vi "Main.vi"() -> ()   [LabVIEW 2017]
panel:
  out "speed":dbl(knob) scale=0.0..10.0
  out "i":i32
  in  "STATUS":string
  in  "stop":bool
  out "ip":string
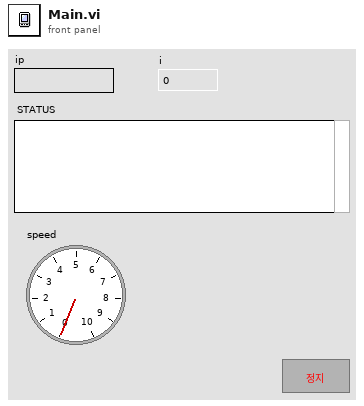
[diagram p1: front panel]
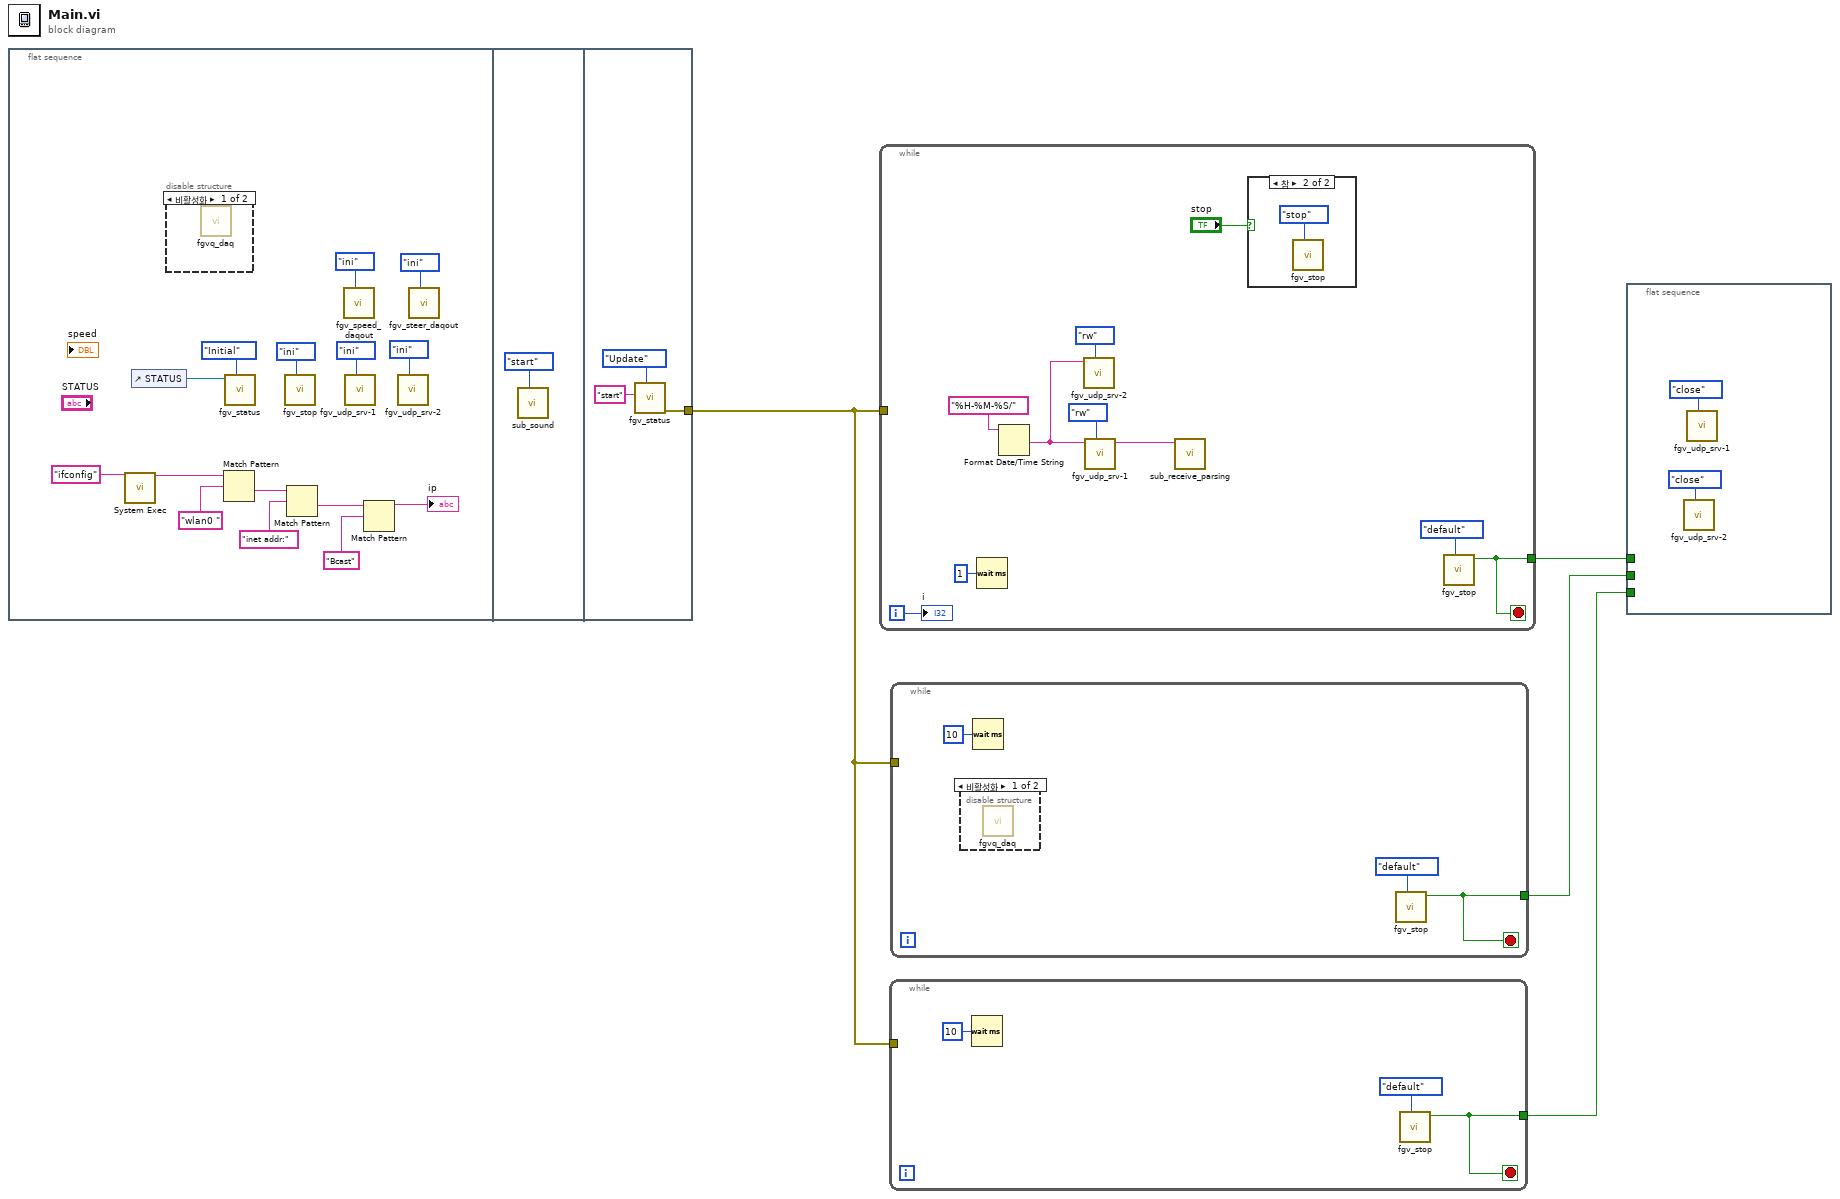
[diagram p0: block diagram]
diagram:
  n1 = flat-sequence {
    tunnel: [w21] -> w1
    frame #0 {
      n2 = call <vilib>:"System Exec.vi"("command line"="ifconfig") -> ("standard output"=w18:string)  [unwired: 7 in, 3 out]
      n3 = control-ref of="STATUS"() -> (w11:refnum<vi>)
      n4 = disable-structure shown="비활성화" {
        frame Disabled {
          n5 = call "fgvq_daq.vi"() -> ()  [unwired: 10 in, 2 out]
        }
        frame Enabled {
        }
      }
      n6 = Match Pattern(string=w18, regular expression="wlan0 ") -> (after substring=w16:string)  [unwired: 1 in, 3 out]
      n7 = call "fgv_status.vi"("Mode"=enum16{"Initial", "Update", "Clear"}."Initial", "System Log"=w11) -> ()  [unwired: 9 in, 1 out]
      n8 = call "fgv_stop.vi"("cmd"=enum16{"default", "ini", "stop"}."ini") -> ()  [unwired: 9 in, 2 out]
      n9 = Match Pattern(string=w16, regular expression="inet addr:") -> (after substring=w14:string)  [unwired: 1 in, 3 out]
      n10 = call "fgv_speed_daqout.vi"("cmd"=enum16{"speed", "close", "ini"}."ini") -> ()  [unwired: 10 in, 1 out]
      n11 = call "fgv_udp_srv-1.vi"("cmd"=enum16{"close", "rw", "ini"}."ini") -> ()  [unwired: 9 in, 2 out]
      n12 = Match Pattern(string=w14, regular expression="Bcast") -> (before substring=→"ip":string)  [unwired: 1 in, 3 out]
      n13 = call "fgv_udp_srv-2.vi"("cmd"=enum16{"close", "rw", "ini"}."ini") -> ()  [unwired: 9 in, 2 out]
      n14 = call "fgv_steer_daqout.vi"("cmd"=enum16{"steer", "close", "ini"}."ini") -> ()  [unwired: 10 in, 1 out]
    }
    frame #1 {
      n15 = call "sub_sound.vi"("cmd"=enum16{"start", "key_lock"}."start") -> ()  [unwired: 10 in, 1 out]
    }
    frame #2 {
      n16 = call "fgv_status.vi"("Mode"=enum16{"Initial", "Update", "Clear"}."Update", "String in"="start") -> ("ERR-OUT"=w21:errorcluster)  [unwired: 9 in]
    }
  }
  n17 = while {
    tunnel: [w26] -> w4
    tunnel: w1 -> [_]
    i -> [w27]
    stop <- w26 stop-if-true
    n18 = Wait (ms)(milliseconds to wait=u32 1 ("대기 시간 (ms)")) -> ()  [unwired: 1 out]
    n19 = Format Date/Time String(time format string (%c)="%H-%M-%S/" ("시간 포맷 문자열 (%c)")) -> (date/time string=w28:string)  [unwired: 2 in]
    n20 = call "fgv_udp_srv-2.vi"("cmd"=enum16{"close", "rw", "ini"}."rw", "data_in"=w28) -> ()  [unwired: 8 in, 2 out]
    n21 = call "fgv_udp_srv-1.vi"("cmd"=enum16{"close", "rw", "ini"}."rw", "data_in"=w28) -> ("data_out"=w24:string)  [unwired: 8 in, 1 out]
    n22 = call "sub_receive_parsing.vi"("data_out 입력"=w24) -> ()  [unwired: 10 in, 1 out]
    n23 = case shown="참" "stop" {
      frame False {
      }
      frame True {
        n24 = call "fgv_stop.vi"("cmd"=enum16{"default", "ini", "stop"}."stop") -> ()  [unwired: 9 in, 2 out]
      }
    }
    n25 = call "fgv_stop.vi"("cmd"=enum16{"default", "ini", "stop"}."default") -> ("stop"=w26:bool)  [unwired: 9 in, 1 out]
    "i" <- w27
  }
  n26 = while {
    tunnel: [w35] -> w2
    tunnel: w1 -> [_]
    stop <- w35 stop-if-true
    n27 = Wait (ms)(milliseconds to wait=u32 10 ("대기 시간 (ms)")) -> ()  [unwired: 1 out]
    n28 = call "fgv_stop.vi"("cmd"=enum16{"default", "ini", "stop"}."default") -> ("stop"=w35:bool)  [unwired: 9 in, 1 out]
  }
  n29 = while {
    tunnel: w1 -> [_]
    tunnel: [w38] -> w3
    stop <- w38 stop-if-true
    n30 = disable-structure shown="비활성화" {
      frame Disabled {
        n31 = call "fgvq_daq.vi"() -> ()  [unwired: 10 in, 2 out]
      }
      frame Enabled {
      }
    }
    n32 = Wait (ms)(milliseconds to wait=u32 10 ("대기 시간 (ms)")) -> ()  [unwired: 1 out]
    n33 = call "fgv_stop.vi"("cmd"=enum16{"default", "ini", "stop"}."default") -> ("stop"=w38:bool)  [unwired: 9 in, 1 out]
  }
  n34 = flat-sequence {
    tunnel: w4 -> [_]
    tunnel: w3 -> [_]
    tunnel: w2 -> [_]
    frame #0 {
      n35 = call "fgv_udp_srv-2.vi"("cmd"=enum16{"close", "rw", "ini"}."close") -> ()  [unwired: 9 in, 2 out]
      n36 = call "fgv_udp_srv-1.vi"("cmd"=enum16{"close", "rw", "ini"}."close") -> ()  [unwired: 9 in, 2 out]
    }
  }
